vi "Latest Parameters.vi"(4 "error in (no error)":errorcluster, 5 "Subject Number":u16, 7 "Subject Parameters Folder":path=path "Z:/Lee Lab/CP FES Walking 2018/Subject Parameters") -> (0 "error in (no error)":errorcluster, 1 "Subject Parameters":T1 {"Subject" items=["Subject 0", "Subject 1", "Subject 2", "Subject 3", "Subject 4", "Subject 5", "Subject 6", "Subject 7", "Subject 8", "Subject 9", "Subject 10", "Subject 11", "Subject 12", "Subject 13", "Subject 14", "Subject 15", "Subject 16", "Subject 17", "Subject 18", "Subject 19", "Subject 20", "Subject 21", "Subject 22", "Subject 23", "Subject 24", "Subject 25", "Subject 26", "Subject 27", "Subject 28", "Subject 29", "Subject 30", "Subject 31", "Subject 32", "Subject 33", "Subject 34", "Subject 35", "Subject 36", "Subject 37", "Subject 38", "Subject 39", "Subject 40"]}, 2 "Source Parameter File":path, 3 "Subject Parameter Folder":path)   [LabVIEW 2019]
uses:
  Controls/Subject Params.ctl
  Controls/Subject.ctl
  Controls/GPD Side Parameters.ctl
  Controls/Type Defs/Stim Parameters.ctl
  Controls/Stim off-half-ful.ctl
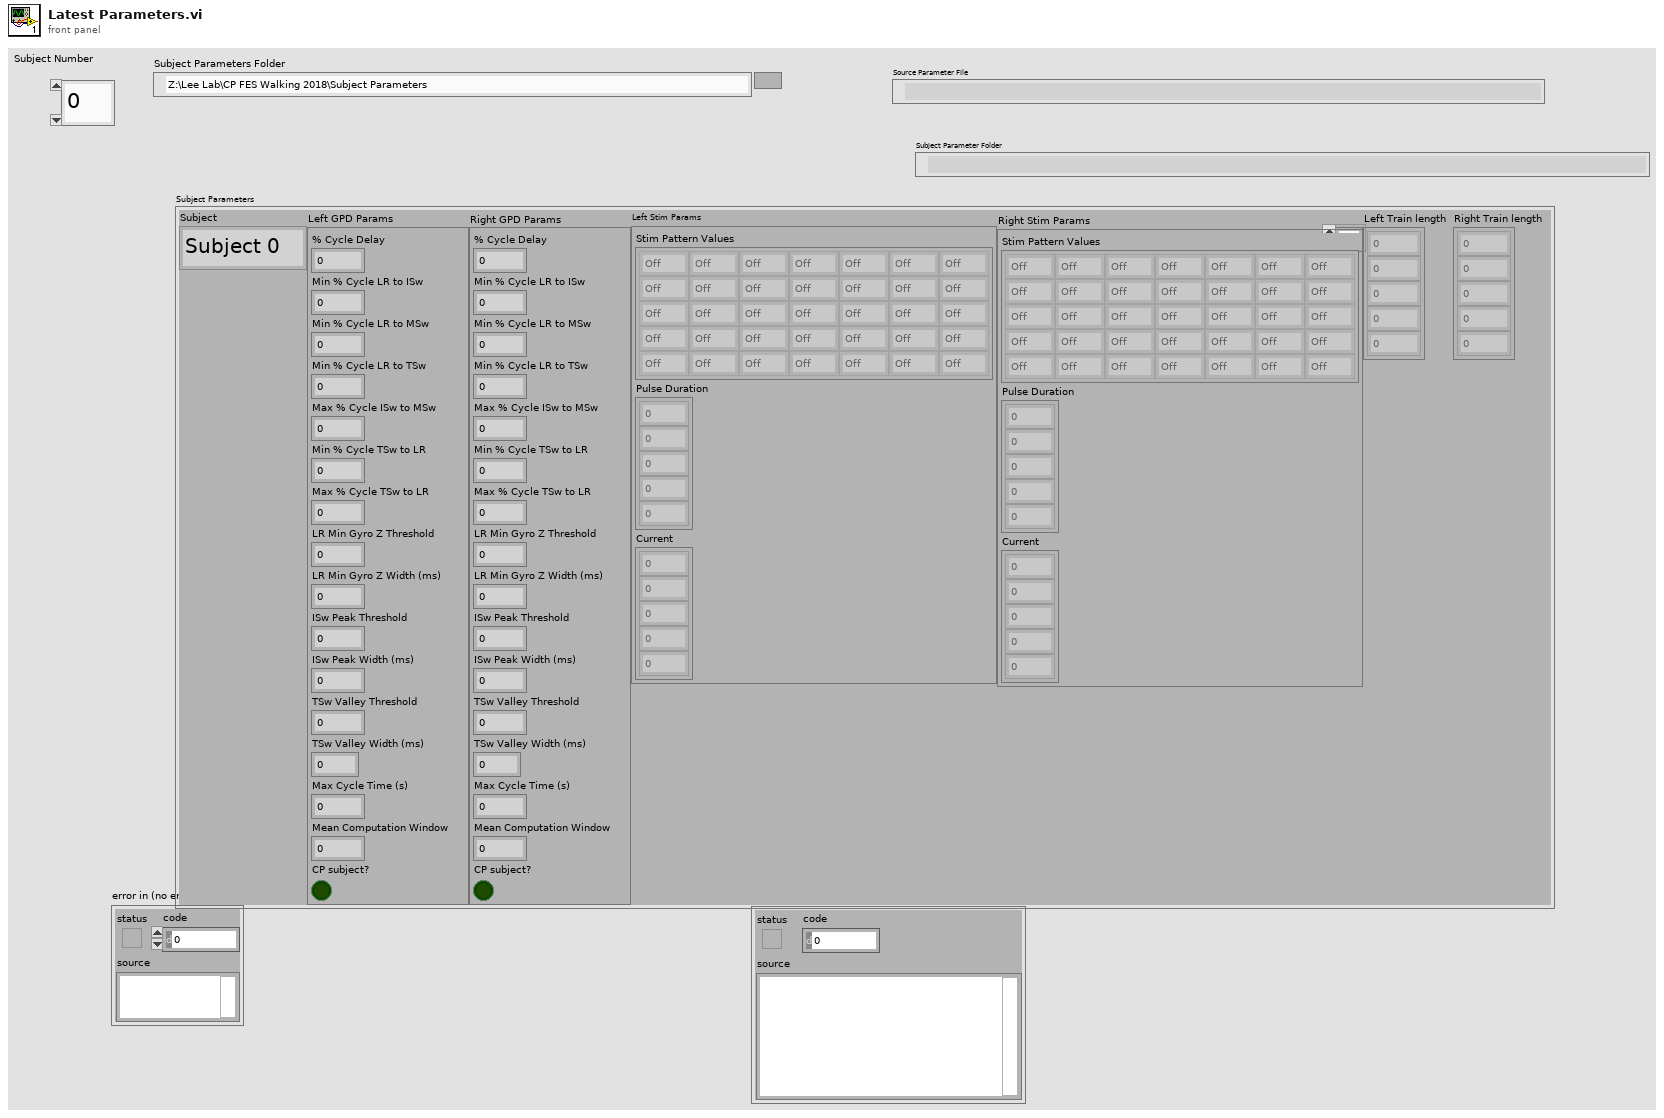
[diagram p1: front panel]
types:
  T1 = typedef "Subject Params.ctl" = cluster{"Subject":T2, "Left GPD Params":T3, "Right GPD Params":T3, "Left Stim Params":T4, "Right Stim Params":T4, "Left Train length":i64[], "Right Train length":i64[]}
  T2 = typedef "Subject.ctl" = u16
  T3 = typedef "GPD Side Parameters.ctl" = cluster{"% Cycle Delay":dbl, "Min % Cycle LR to ISw ":dbl, "Min % Cycle LR to MSw":dbl, "Min % Cycle LR to TSw":dbl, "Max % Cycle ISw to MSw":dbl, "Min % Cycle TSw to LR":dbl, "Max % Cycle TSw to LR":dbl, "LR Min Gyro Z Threshold":dbl, "LR Min Gyro Z Width":dbl, "ISw Peak Threshold":dbl, "ISw Peak Width":dbl, "TSw Valley Threshold":dbl, "TSw Valley Width (ms)":dbl, "Max Cycle Time (s)":dbl, "Mean Computation Window":dbl, "CP subject?":bool}
  T4 = typedef "Stim Parameters.ctl" = cluster{"Stim Pattern Values":T5[][], "Pulse Duration":i64[], "Current":i64[]}
  T5 = typedef "Stim off-half-ful.ctl" = enum16{"Off", "Half", "Full"}
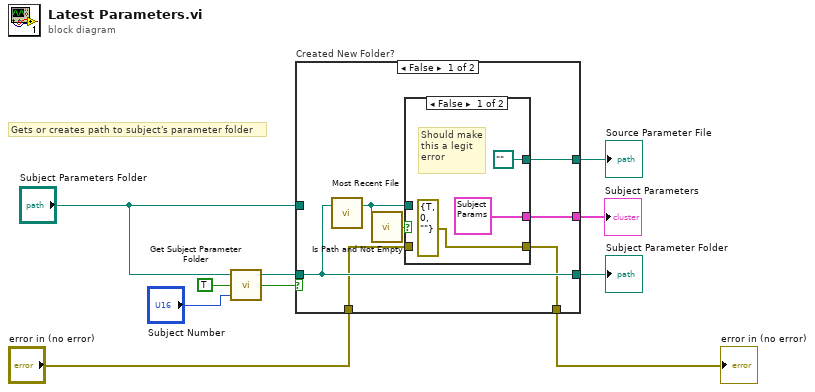
[diagram p0: block diagram]
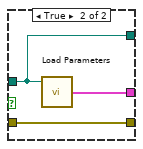
[diagram p2: hidden frame]
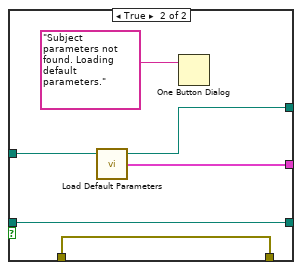
[diagram p3: hidden frame]
diagram:
  # "Gets or creates path to subject's parameter folder"
  n1 = call "Get Subject Parameter Folder.vi"("Subject Number"="Subject Number", "Create if DNE?"=TRUE, "Subject Parameter Path"="Subject Parameters Folder") -> ("Created new?"=w8:bool, "Subject Parameter Folder"=w6:path)  [unwired: 1 out]
  n2 = case "Created New Folder?" shown="False" w8 {
    tunnel: "Subject Parameters Folder" -> [_ w29]
    tunnel: w6 -> [w16 w27]
    tunnel: [w17 w28] -> w5
    tunnel: [w16 w27] -> w4
    tunnel: [w13 w25] -> w3
    tunnel: [w12 w24] -> w2
    tunnel: "error in (no error)" -> [w11 w24]
    frame False {
      n3 = call "Most Recent File.vi"("Folder Path In"=w16) -> ("File Path Out"=w15:path)  [unwired: 1 in, 1 out]
      n4 = call <vilib>:"Is Path and Not Empty.vi"("path"=w15) -> ("Is Path and Not Empty?"=w14:bool)  [unwired: 4 in]
      n5 = case shown="False" w14 {
        tunnel: [T1 {"Subject"=0, "Left GPD Params"={"% Cycle Delay"=0.0, "Min % Cycle LR to ISw "=0.0, "Min % Cycle LR to MSw"=0.0, "Min % Cycle LR to TSw"=0.0, "Max % Cycle ISw to MSw"=0.0, "Min % Cycle TSw to LR"=0.0, "Max % Cycle TSw to LR"=0.0, "LR Min Gyro Z Threshold"=0.0, "LR Min Gyro Z Width"=0.0, "ISw Peak Threshold"=0.0, "ISw Peak Width"=0.0, "TSw Valley Threshold"=0.0, "TSw Valley Width (ms)"=0.0, "Max Cycle Time (s)"=0.0, "Mean Computation Window"=0.0, "CP subject?"=FALSE}, "Right GPD Params"={"% Cycle Delay"=0.0, "Min % Cycle LR to ISw "=0.0, "Min % Cycle LR to MSw"=0.0, "Min % Cycle LR to TSw"=0.0, "Max % Cycle ISw to MSw"=0.0, "Min % Cycle TSw to LR"=0.0, "Max % Cycle TSw to LR"=0.0, "LR Min Gyro Z Threshold"=0.0, "LR Min Gyro Z Width"=0.0, "ISw Peak Threshold"=0.0, "ISw Peak Width"=0.0, "TSw Valley Threshold"=0.0, "TSw Valley Width (ms)"=0.0, "Max Cycle Time (s)"=0.0, "Mean Computation Window"=0.0, "CP subject?"=FALSE}, "Left Stim Params"={"Stim Pattern Values"=[], "Pulse Duration"=[], "Current"=[]}, "Right Stim Params"={"Stim Pattern Values"=[], "Pulse Duration"=[], "Current"=[]}, "Left Train length"=[], "Right Train length"=[]} ("Subject Parameters") w23] -> w17
        tunnel: w15 -> [_ w22]
        tunnel: [path "" ("File Path Out") w22] -> w13
        tunnel: [errorcluster {"status"=TRUE, "code"=0, "source"=""} ("error constant") w21] -> w12
        tunnel: w11 -> [_ w21]
        frame False {
          # "Should make this a legit error"
        }
        frame True {
          n6 = call "Load Parameters.vi"("Subject Parameters File"=w22) -> ("Subject Parameters"=w23:T1)  [unwired: 2 in, 2 out]
        }
      }
    }
    frame True {
      n7 = call "Load Default Parameters.vi"("Default parameters file"=w29) -> ("Subject Parameters"=w28:T1, "Subject Parameters File"=w25:path)  [unwired: 3 in]
      n8 = One Button Dialog(message="Subject parameters not found. Loading default parameters.") -> ()  [unwired: 1 in, 1 out]
    }
  }
  "error in (no error)" <- w2
  "Subject Parameters" <- w5
  "Subject Parameter Folder" <- w4
  "Source Parameter File" <- w3
